vi "Cleanup.vi"(8 "error in (no error)":errorcluster, 11 "GWebAppArrayPanel in":refnum<class "GWebAppArrayPanel.lvclass">) -> (0 "error out":errorcluster)   [LabVIEW 2020, in "PicoG-App.lvlib" / "GWebAppArrayPanel.lvclass"]
uses:
  GWebAppArrayPanel.lvclass
  GWebAppArrayPanel.lvclass/GWebAppArrayPanel.ctl
  <vilib>/IlluminatedG/IG OOPanel/OOPanel/ArrayPanel/ArrayPanel.lvclass
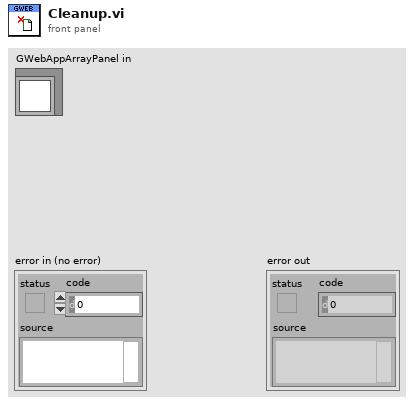
[diagram p1: front panel]
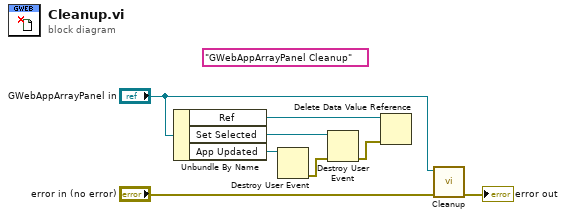
[diagram p0: block diagram]
diagram:
  (unwired) "GWebAppArrayPanel Cleanup" ("message")
  n1 = Unbundle By Name("GWebAppArrayPanel in") -> ("Ref"=w2:refnum<data-value>, "Set Selected"=w4:refnum<user-event>, "App Updated"=w5:refnum<user-event>)
  n2 = Destroy User Event(user event=w5) -> (error out=w3:errorcluster)  [unwired: 1 in]
  n3 = Destroy User Event(user event=w4, error in=w3) -> (error out=w1:errorcluster)
  n4 = Delete Data Value Reference(data value reference=w2, error in=w1) -> ()  [unwired: 2 out]
  n5 = call-parent "Cleanup.vi"("error in (no error)"="error in (no error)", "ArrayPanel in"="GWebAppArrayPanel in") -> ("error out"=→"error out":errorcluster)  [unwired: 9 in]
